vi "Select Prism.vi"(8 "error in (no error)":errorcluster {"code" format="%.0x"}, 9 "Prism Position (0: Bi)":enum16{"Bi", "Side"}(ring), 10 "Device Number (1)":i32=1, 11 "VISA Resource Name":refnum<visa-resource-name>) -> (0 "error out":errorcluster {"code" format="%.0x"}, 3 "VISA Resource Name Out":refnum<visa-resource-name>)   [LabVIEW 2020, in "Olympus IX BX Series.lvlib"]
doc: "Engages the specified prism in the light axis.\n\nNotes:\n(1) This VI is valid only for Olympus IX2 model."
uses:
  Olympus IX BX Series.lvlib
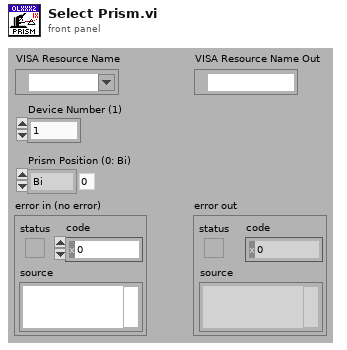
[diagram p1: front panel]
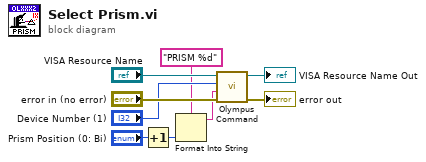
[diagram p0: block diagram]
diagram:
  n1 = Increment(x="Prism Position (0: Bi)") -> (x+1=w1:enum16{"Bi", "Side"})
  n2 = Format Into String(format string="PRISM %d", w1) -> (resulting string=w6:string)  [unwired: 2 in, 1 out]
  n3 = call "Olympus Command.vi"("error in (no error)"="error in (no error)", "Command string"=w6, "Device Number (1)"="Device Number (1)", "VISA Resource Name"="VISA Resource Name") -> ("error out"=→"error out":errorcluster, "VISA Resource Name Out"=→"VISA Resource Name Out":refnum<visa-resource-name>)  [unwired: 5 in, 1 out]
